vi "Insert Instrument Class by Name.vi"(8 "error in (no error)":errorcluster, 9 "Type":T1, 10 "Instrument in":refnum<class "Instrument.lvclass">, 11 "Control Experiment in":refnum<class "Control Experiment.lvclass">) -> (0 "error out":errorcluster, 1 "Found?":bool, 2 "Instrument out":refnum<class "Instrument.lvclass">, 3 "Control Experiment out":refnum<class "Control Experiment.lvclass">)   [LabVIEW 2019, in "Control Experiment.lvclass"]
uses:
  Control Experiment.lvclass
  Typedefs/Instrument Types--enum.ctl
  <userlib>/LevyLab/Instrument Framework/Instrument/Instrument.lvclass
  Control Experiment.lvclass/Control Experiment.ctl
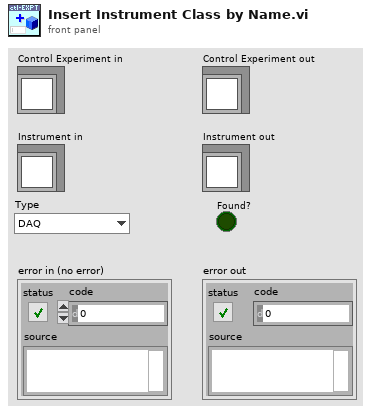
[diagram p1: front panel]
types:
  T1 = typedef "Control Experiment.lvclass/Instrument Types--enum.ctl" = enum16{"DAQ", "Amplifier", "Temperature", "Magnet", "Rotator", "Level", "Capacitance", "Delay Line", "Strain Cell", "VNA", "Source"}
  T2 = typedef "Control Experiment.lvclass/Instrument Classes--cluster.ctl" = cluster{"DAQ":refnum<class "Instrument.LockinAPI.lvclass">, "Amplifier":refnum<class "Instrument.Amplifier.lvclass">, "Temperature":refnum<class "Instrument.Cryostat.lvclass">, "Magnet":refnum<class "Instrument.Cryostat.lvclass">, "Rotator":refnum<class "Instrument.Cryostat.lvclass">, "Level":refnum<class "Instrument.Cryostat.lvclass">, "Capacitance":refnum<class "Instrument.CBridge.lvclass">, "Delay Line":refnum<class "Instrument.DelayLine.lvclass">, "Strain Cell":refnum<class "Instrument.Strain.lvclass">, "VNA":refnum<class "Instrument.VNA.lvclass">, "Source":refnum<class "Instrument.VSource.lvclass">}
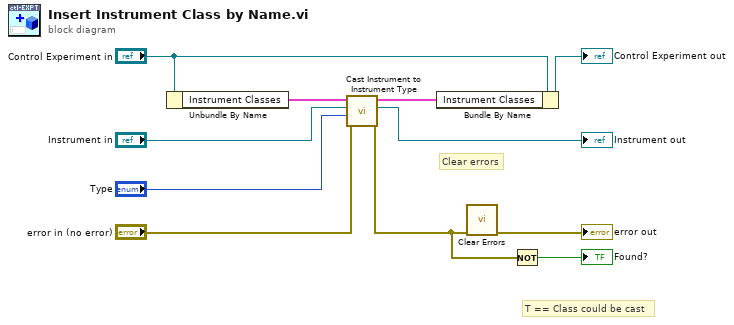
[diagram p0: block diagram]
diagram:
  # "T == Class could be cast"
  # "Clear errors"
  n1 = Unbundle By Name("Control Experiment in") -> ("Instrument Classes"=w7:T2)
  n2 = call "Cast Instrument to Instrument Type.vi"("error in (no error)"="error in (no error)", "Type"="Type", "Instrument in"="Instrument in", "Instrument Classes"=w7) -> ("error out"=w4:errorcluster, "Instrument out"=→"Instrument out":refnum<class "Instrument.lvclass">, "Instrument Classes out"=w6:T2)  [unwired: 5 in]
  n3 = Bundle By Name(cluster="Control Experiment in", "Instrument Classes"=w6) -> (→"Control Experiment out":refnum<class "Control Experiment.lvclass">)
  n4 = call <vilib>:"Clear Errors.vi"("error in (no error)"=w4) -> ("error out"=→"error out":errorcluster)  [unwired: 5 in, 1 out]
  n5 = Not(x=w4) -> (.not. x?=→"Found?":bool)
